vi "DeCoF UDP broadcast identification.vi"(4 "timeout ms (25000)":i32=1000, 6 "error in (no error)":errorcluster, 7 "sender ID":string="LabVIEW", 8 "port":u16=60010) -> (0 "error out":errorcluster, 1 "ip-addresses":string[](array[string]), 2 "number":i32, 3 "device list":T1(array[cluster]), 5 "serials and IPs":string[][](array[string]))   [LabVIEW 2013]
doc: "This VI scans the local network for available TOPTICA lasers. It sends an UDP broadcast to all network addresses on port 60003. The lasers detect the broadcast and send back a telegram with their serial number and their IP number. The VI collects all these replies and returns an array with the resulting list."
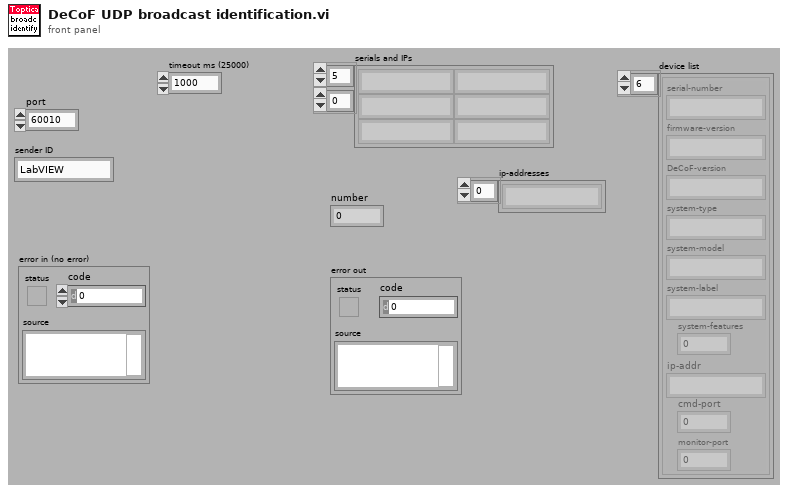
[diagram p1: front panel]
types:
  T1 = cluster{"serial-number":string, "firmware-version":string, "DeCoF-version":string, "system-type":string, "system-model":string, "system-label":string, "system-features":i32, "ip-addr":string, "cmd-port":i32, "monitor-port":i32}[]
  T2 = cluster{"serial-number":string, "firmware-version":string, "DeCoF-version":string, "system-type":string, "system-model":string, "system-label":string, "system-features":i32, "ip-addr":string, "cmd-port":i32, "monitor-port":i32}
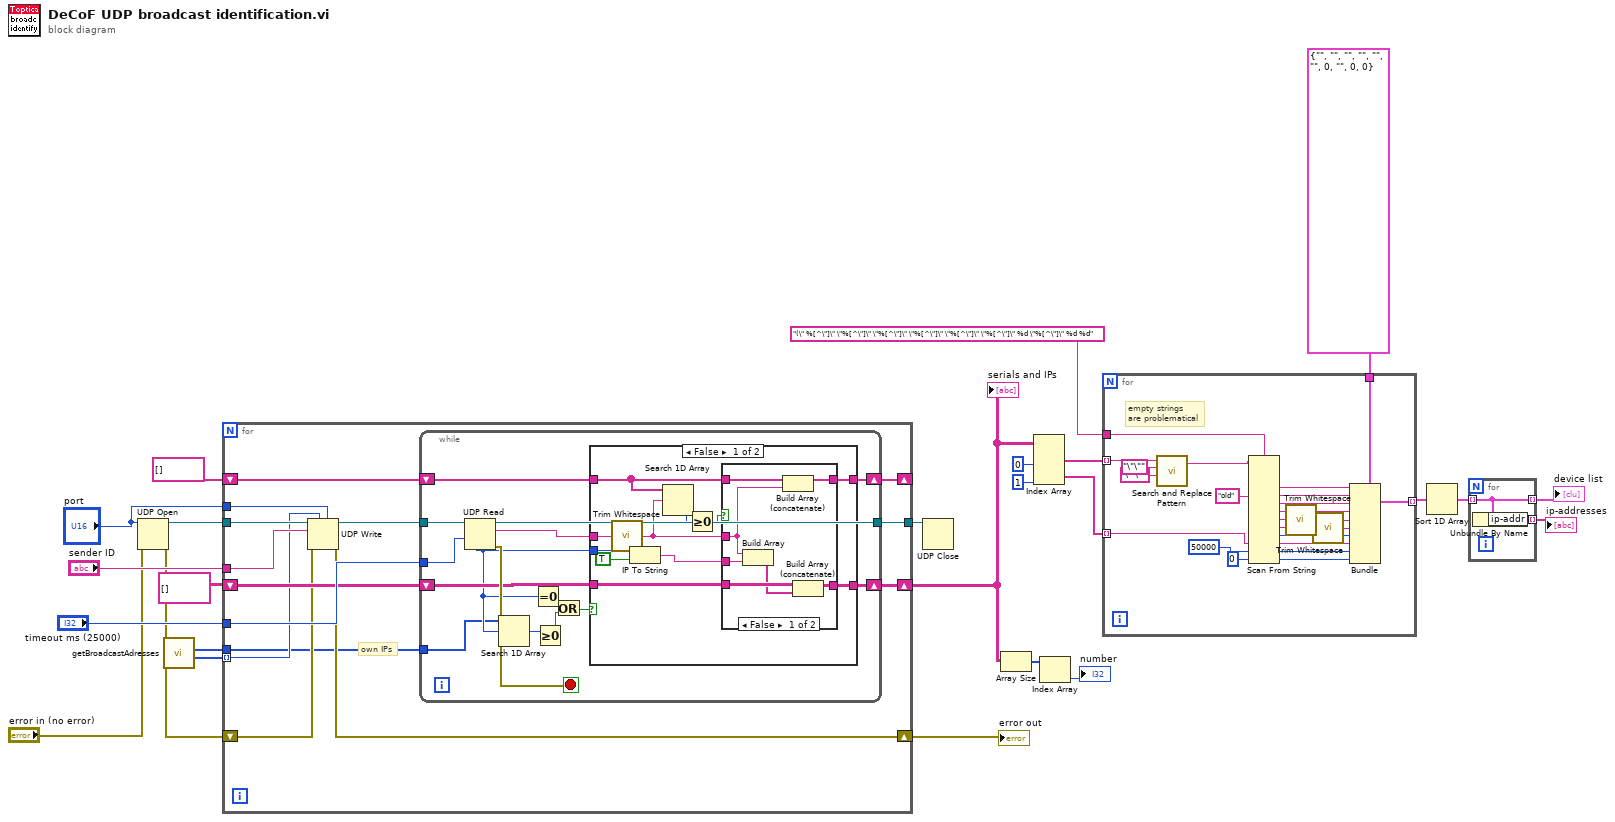
[diagram p0: block diagram]
diagram:
  n1 = UDP Open(8:"error in (no error)", 11:"port") -> (port=w23:refnum<k16>, 0:w15:errorcluster)  [unwired: 3 in, 1 out]
  n2 = call "getBroadcastAdresses.vi"() -> ("broadcast addresses"=w16:u32[], "IP addresses"=w14:u32[])  [unwired: 4 in, 2 out]
  n3 = for {
    tunnel: "port" -> [w39]
    tunnel: "sender ID" -> [w38]
    tunnel: w23 -> [w36]
    tunnel: "timeout ms (25000)" -> [w35]
    tunnel: [w34] -> w18
    shift-right: [w33] -> w5
    shift-left: string[][] [] -> [w32]
    tunnel: w16 -> [w29] mode=indexing
    shift-right: [w30] -> w13
    shift-left: w15 -> [w31]
    tunnel: w14 -> [w28]
    shift-right: [w26] -> _
    shift-left: string[] [] -> [w27]
    # "own IPs"
    n4 = UDP Write(address=w29, port or service name=w39, connection ID=w36, data in=w38, 8:w31) -> (error out=w30:errorcluster, 3:w37:refnum<k16>)  [unwired: 1 in]
    n5 = while {
      tunnel: w37 -> [w54]
      shift-right: [w50] -> w33
      shift-left: w32 -> [w51]
      tunnel: w35 -> [w47]
      tunnel: [w46] -> w34
      tunnel: w28 -> [w42]
      shift-right: [w40] -> w26
      shift-left: w27 -> [w41]
      stop <- w53 stop-if-true
      n6 = UDP Read(connection ID=w54, timeout ms (25000)=w47) -> (data out=w52:string, error out=w53:errorcluster, 3:w46:refnum<k16>, 6:w45:u32)  [unwired: 2 in, 1 out]
      n7 = Search 1D Array(1D array=w42, element=w45) -> (index of element=w44:i32)  [unwired: 1 in]
      n8 = Equal To 0?(x=w45) -> (x = 0?=w49:bool)
      n9 = Greater Or Equal To 0?(x=w44) -> (x >= 0?=w43:bool)
      n10 = Or(x=w49, y=w43) -> (x .or. y?=w48:bool)
      n11 = case shown="False" w48 {
        tunnel: w52 -> [w64 _]
        tunnel: w51 -> [w62 w76]
        tunnel: [w61 w76] -> w50
        tunnel: w45 -> [w60 _]
        tunnel: w41 -> [w59 w75]
        tunnel: [w58 w75] -> w40
        frame False {
          n12 = call <vilib>:"Trim Whitespace.vi"("string"=w64) -> ("trimmed string"=w57:string)  [unwired: 1 in]
          n13 = IP To String(1:TRUE ("dot notation? (F)"), 2:w60) -> (0:w63:string)
          n14 = Search 1D Array(1D array=w59, element=w57) -> (index of element=w55:i32)  [unwired: 1 in]
          n15 = Greater Or Equal To 0?(x=w55) -> (x >= 0?=w56:bool)
          n16 = case shown="False" w56 {
            tunnel: w63 -> [w72 _]
            tunnel: w62 -> [w71 w73]
            tunnel: [w69 w73] -> w61
            tunnel: w59 -> [w68 w74]
            tunnel: [w67 w74] -> w58
            tunnel: w57 -> [w66 _]
            frame False {
              n17 = Build Array(w66, w72) -> (w70:string[])
              n18 = Build Array (concatenate)(w68, w66) -> (w67:string[])
              n19 = Build Array (concatenate)(w71, w70) -> (w69:string[][])
            }
            frame True {
              # "avoid\nduplicates"
            }
          }
        }
        frame True {
        }
      }
    }
  }
  "error out" <- w13
  "serials and IPs" <- w5
  n20 = UDP Close(connection ID=w18) -> ()  [unwired: 1 in, 2 out]
  n21 = Array Size(array=w5) -> (size(s)=w20:i32[])
  n22 = Index Array(array=w5, index (col) #1=0 ("disabled index (col)"), index (col) #2=1 ("index (col)")) -> (element #1=w9:string[], element #2=w8:string[])  [unwired: 2 in]
  n23 = Index Array(array=w20) -> (element=→"number":i32)  [unwired: 1 in]
  n24 = for {
    tunnel: w9 -> [w84] mode=indexing
    tunnel: w8 -> [w86] mode=indexing
    tunnel: [w96] -> w4 mode=indexing
    tunnel: "(\" %[^\"]\" \"%[^\"]\" \"%[^\"]\" \"%[^\"]\" \"%[^\"]\" \"%[^\"]\" %d \"%[^\"]\" %d %d" ("format string") -> [w95]
    tunnel: T2 {"serial-number"="", "firmware-version"="", "DeCoF-version"="", "system-type"="", "system-model"="", "system-label"="", "system-features"=0, "ip-addr"="", "cmd-port"=0, "monitor-port"=0} -> [w94]
    # "empty strings\nare problematical"
    n25 = call <vilib>:"Search and Replace Pattern.vi"("string"=w84, "regular expression (\"\")"="\"\"" ("regular expression (\"\")"), "replace string (\"\")"="\" \"" ("replace string (\"\")")) -> ("result string"=w81:string)  [unwired: 2 in, 1 out]
    n26 = Scan From String(format string=w95, input string=w81, default 2="old" ("element"), default 8=w86, default 9=50000 ("default value 9"), default 10=0 ("default value 10")) -> (output 1=w99:string, output 2=w98:string, output 3=w97:string, output 4=w93:string, output 5=w80:string, output 6=w79:string, output 7=w88:i32, output 8=w87:string, output 9=w89:i32, output 10=w90:i32)  [unwired: 8 in, 3 out]
    n27 = call <vilib>:"Trim Whitespace.vi"("string"=w80) -> ("trimmed string"=w77:string)  [unwired: 1 in]
    n28 = call <vilib>:"Trim Whitespace.vi"("string"=w79) -> ("trimmed string"=w78:string)  [unwired: 1 in]
    n29 = Bundle(cluster=w94, "serial-number"=w99, "firmware-version"=w98, "DeCoF-version"=w97, "system-type"=w93, "system-model"=w77, "system-label"=w78, "system-features"=w88, "ip-addr"=w87, "cmd-port"=w89, "monitor-port"=w90) -> (w96:T2)
  }
  n30 = Sort 1D Array(array=w4) -> (sorted array=w3:T1)
  n31 = for {
    tunnel: w3 -> [w101] mode=indexing
    tunnel: [w101] -> w2 mode=indexing
    tunnel: [w100] -> w1 mode=indexing
    n32 = Unbundle By Name(w101) -> ("ip-addr"=w100:string)
  }
  "device list" <- w2
  "ip-addresses" <- w1
